vi "Job Done.vi"(8 "error in (no error)":errorcluster, 10 "Job":refnum<class "Job.lvclass">, 11 "Jobber in":refnum<class "Jobber.lvclass">) -> (0 "error out":errorcluster, 3 "Jobber out":refnum<class "Jobber.lvclass">)   [LabVIEW 2014, in "Jobber.lvlib" / "Jobber.lvclass"]
uses:
  Jobber.lvclass
  Classes/Job/Job.lvclass
  Jobber.lvclass/Jobber.ctl
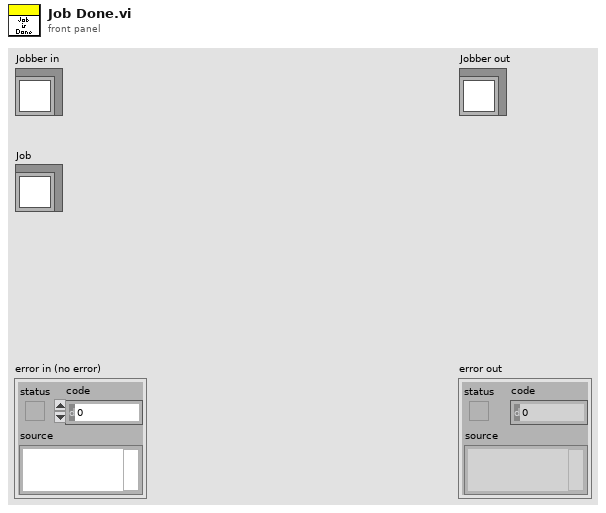
[diagram p1: front panel]
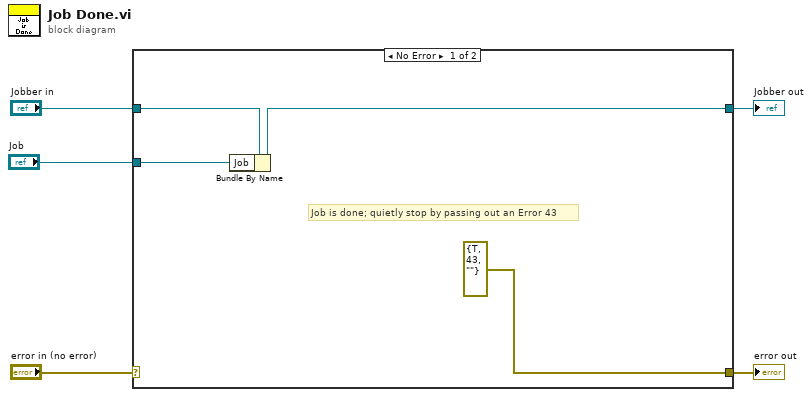
[diagram p0: block diagram]
diagram:
  n1 = case shown="No Error" "error in (no error)" {
    selector: "error in (no error)" -> [_ w11]
    tunnel: [errorcluster {"status"=TRUE, "code"=43, "source"=""} ("error in") w11] -> w4
    tunnel: [w7 w10] -> w2
    tunnel: "Jobber in" -> [w9 w10]
    tunnel: "Job" -> [w8 _]
    frame No Error {
      # "Job is done; quietly stop by passing out an Error 43"
      n2 = Bundle By Name(cluster=w9, "Job"=w8) -> (w7:refnum<class "Jobber.lvclass">)
    }
    frame Error {
    }
  }
  "error out" <- w4
  "Jobber out" <- w2
